vi "Code Alphabet.vi"() -> (2 "Code Alphabet":string="~-_.0123456789abcdefghijklmnopqrstuvwxyzABCDEFGHIJKLMNOPQRSTUVWXYZ")   [LabVIEW 2020, in "OAuth2.lvlib"]
uses:
  OAuth2.lvlib
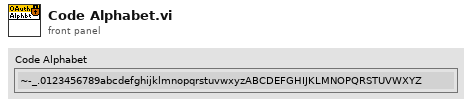
[diagram p1: front panel]
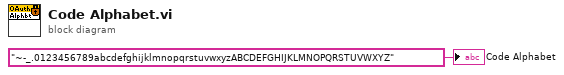
[diagram p0: block diagram]
diagram:
  "Code Alphabet" <- "~-_.0123456789abcdefghijklmnopqrstuvwxyzABCDEFGHIJKLMNOPQRSTUVWXYZ" ("Alphabet (Default)")
